vi "__FpCtrlType.vi"(8 "error out":errorcluster, 11 "reference":refnum<vi>) -> (0 "error out 2":errorcluster, 1 "ControlsIndicator":refnum<vi>[](array[refnum]), 2 "Controls":refnum<vi>[](array[refnum]), 3 "reference (dup)":refnum<vi>)   [LabVIEW 2017]
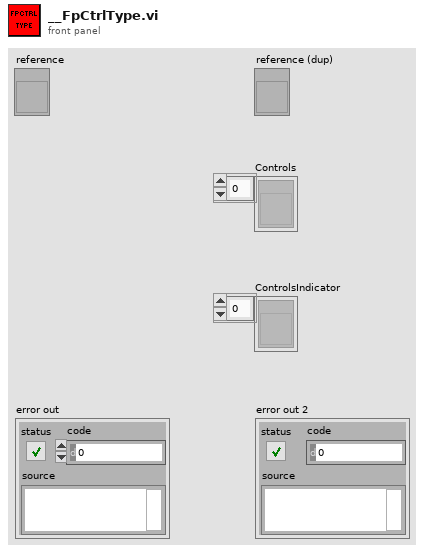
[diagram p1: front panel]
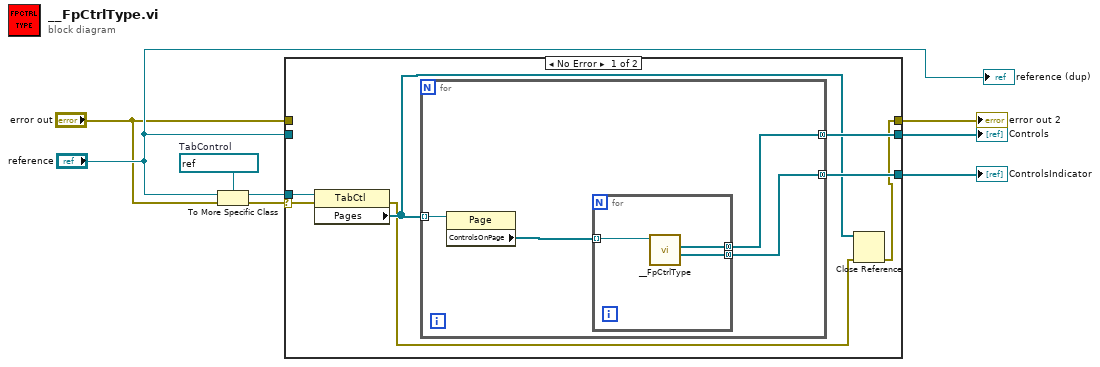
[diagram p0: block diagram]
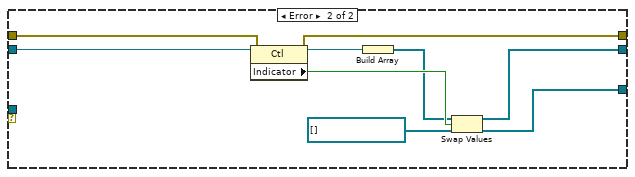
[diagram p2: hidden frame]
diagram:
  w8 = refnum<vi> refnum  # TabControl
  n1 = To More Specific Class(target class=w8, reference="reference", error in="error out") -> (specific class reference=w6:refnum<vi>, error out=w7:errorcluster)
  n2 = case shown="No Error" w7 {
    selector: w7 -> [w12 _]
    tunnel: [w14 w26] -> w4
    tunnel: "error out" -> [_ w30]
    tunnel: [w9 w29] -> w5
    tunnel: "reference" -> [_ w28]
    tunnel: w6 -> [w15 _]
    tunnel: [w13 w25] -> w3
    frame No Error {
      n3 = property class="TabCtl"(reference=w15, error in=w12) -> (error out=w10:errorcluster, "Pages"=w11:refnum<vi>[])  [unwired: 1 out]
      n4 = for {
        tunnel: w11 -> [w19] mode=indexing
        tunnel: [w18] -> w14 mode=concatenating
        tunnel: [w17] -> w13 mode=concatenating
        n5 = property class="Page"(reference=w19) -> ("ControlsOnPage"=w16:refnum<vi>[])  [unwired: 1 in, 2 out]
        n6 = for {
          tunnel: [w22] -> w18 mode=concatenating
          tunnel: [w21] -> w17 mode=concatenating
          tunnel: w16 -> [w20] mode=indexing
          n7 = call "__FpCtrlType.vi"("reference"=w20) -> ("ControlsIndicator"=w21:refnum<vi>[], "Controls"=w22:refnum<vi>[])  [unwired: 7 in, 2 out]
        }
      }
      n8 = Close Reference(reference=w11, error in (no error)=w10) -> (error out=w9:errorcluster)
    }
    frame Error {
      n9 = property class="Ctl"(reference=w28, error in=w30) -> (reference out=w31:refnum<vi>, error out=w29:errorcluster, "Indicator"=w27:bool)
      n10 = Build Array(w31) -> (w23:refnum<vi>[])
      n11 = Swap Values(12:w23, 13:w27, 14:refnum<vi>[] [] ("appended array")) -> (1:w26:refnum<vi>[], 3:w25:refnum<vi>[])
    }
  }
  "error out 2" <- w5
  "Controls" <- w4
  "ControlsIndicator" <- w3
  "reference (dup)" <- "reference"
